vi "GenerateCode.vi"(0 "XRef":T17, 1 "Terms":T14, 2 "Diagram":T13, 3 "State In":T1) -> (14 "Generated Code?":T9, 15 "Reply":T12, 16 "Fatal Error Out":T11, 17 "State Out":T1)   [LabVIEW 2021, in "myRIO PWM Open.xnode"]
uses:
  <vilib>/myRIO/Instrument Drivers/Onboard IO/PWM/vis/myRIO PWM Open.xnode
  <vilib>/XNodeSupport/XNodeXNodeRef.ctl
  <vilib>/XNodeSupport/XNodeTermIDPairs.ctl
  <vilib>/XNodeSupport/XNodeTermIDPair.ctl
  <vilib>/XNodeSupport/XNodeTermRef.ctl
  <vilib>/XNodeSupport/XNodeString.ctl
  <vilib>/XNodeSupport/XNodeTopLevelDiagramRef.ctl
  <vilib>/myRIO/Instrument Drivers/Onboard IO/PWM/vis/State.ctl
  <vilib>/myRIO/Common/Instrument Driver Framework/Utilities/typedefs/myRIOXPeripheral.ctl
  <vilib>/XNodeSupport/XNodeTerm4Array.ctl
  <vilib>/XNodeSupport/XNodeTerm4.ctl
  <vilib>/XNodeSupport/XNodeVariant.ctl
  <vilib>/XNodeSupport/XNodeRect32.ctl
  <vilib>/XNodeSupport/XNodeInt.ctl
  <vilib>/XNodeSupport/XNodeBool.ctl
  <vilib>/XNodeSupport/XNodeTermDirection.ctl
  <vilib>/XNodeSupport/XNodeStringArray.ctl
  <vilib>/XNodeSupport/XNodeErrorCluster.ctl
  <vilib>/userdefined/High Color/nirio_resource_hc.ctl
  <vilib>/XNodeSupport/NI_XNodeSupport.lvlib
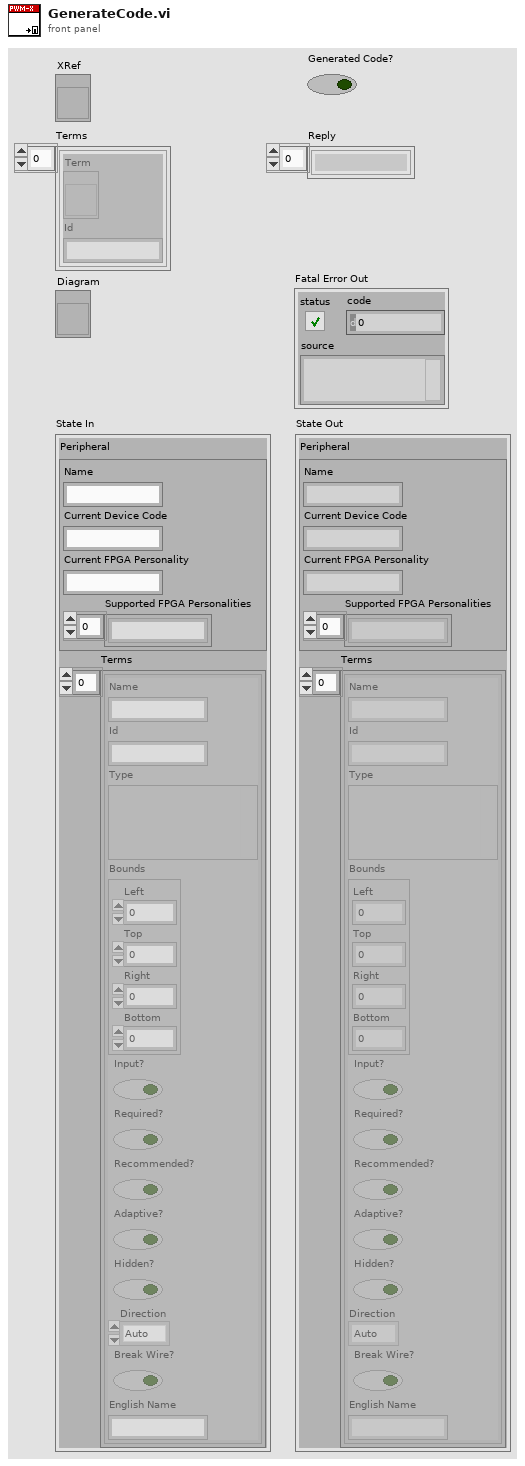
[diagram p1: front panel]
types:
  T1 = typedef "myRIO PWM Open.xnode/State.ctl" = cluster{"Peripheral":T2, "Terms":T3}
  T2 = typedef "myRIOXPeripheral.ctl" = cluster{"Name":string, "Current Device Code":string, "Current FPGA Personality":string, "Supported FPGA Personalities":string[]}
  T3 = typedef "NI_XNodeSupport.lvlib/XNodeTerm4Array.ctl" = T4[]
  T4 = typedef "NI_XNodeSupport.lvlib/XNodeTerm4.ctl" = cluster{"Name":T5, "Id":T5, "Type":T6, "Bounds":T7, "Input?":T9, "Required?":T9, "Recommended?":T9, "Adaptive?":T9, "Hidden?":T9, "Direction":T10, "Break Wire?":T9, "English Name":T5}
  T5 = typedef "NI_XNodeSupport.lvlib/XNodeString.ctl" = string
  T6 = typedef "NI_XNodeSupport.lvlib/XNodeVariant.ctl" = variant
  T7 = typedef "NI_XNodeSupport.lvlib/XNodeRect32.ctl" = cluster{"Left":T8, "Top":T8, "Right":T8, "Bottom":T8}
  T8 = typedef "NI_XNodeSupport.lvlib/XNodeInt.ctl" = i32
  T9 = typedef "NI_XNodeSupport.lvlib/XNodeBool.ctl" = bool
  T10 = typedef "NI_XNodeSupport.lvlib/XNodeTermDirection.ctl" = enum32{"Auto", "Up", "Down", "Left", "Right", "Center"}
  T11 = typedef "NI_XNodeSupport.lvlib/XNodeErrorCluster.ctl" = errorcluster
  T12 = typedef "NI_XNodeSupport.lvlib/XNodeStringArray.ctl" = T5[]
  T13 = typedef "NI_XNodeSupport.lvlib/XNodeTopLevelDiagramRef.ctl" = refnum<vi>
  T14 = typedef "NI_XNodeSupport.lvlib/XNodeTermIDPairs.ctl" = T15[]
  T15 = typedef "NI_XNodeSupport.lvlib/XNodeTermIDPair.ctl" = cluster{"Term":T16, "Id":T5}
  T16 = typedef "NI_XNodeSupport.lvlib/XNodeTermRef.ctl" = refnum<vi>
  T17 = typedef "NI_XNodeSupport.lvlib/XNodeXNodeRef.ctl" = refnum<vi>
  T18 = typedef "nirio_resource_hc.ctl" = tag
  T19 = typedef "LVPositionTypeDef.ctl" = cluster{"Left":i32, "Top":i32}
  T20 = typedef "Hardware Version Enum.ctl" = enum16{"Unknown", "myRIO-1900", "myRIO-1950", "roboRIO", "NI ELVIS RIO CM", "ELVIS III"}
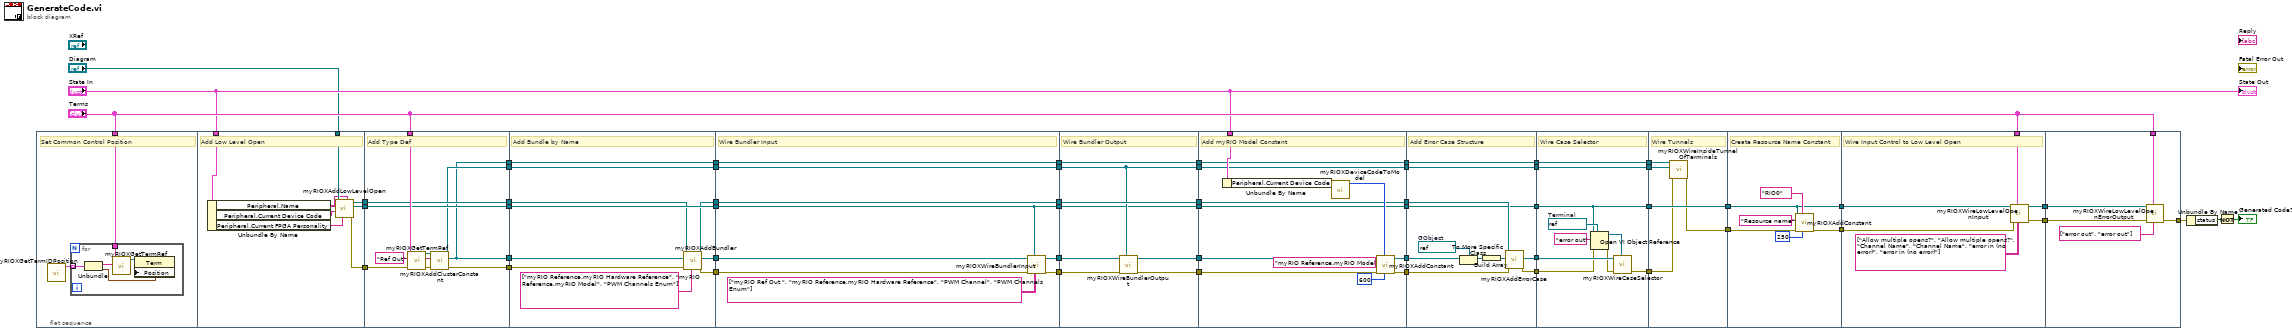
[diagram p0: block diagram]
diagram:
  n1 = flat-sequence {
    tunnel: "Terms" -> [w56]
    tunnel: "State In" -> [w69]
    tunnel: "Diagram" -> [w68]
    tunnel: [w67] -> w52
    tunnel: [w66] -> w48
    tunnel: [w64] -> w14
    tunnel: "Terms" -> [w79]
    tunnel: [w73] -> w54
    tunnel: [w76] -> w53
    tunnel: w52 -> [w76]
    tunnel: [w75] -> w49
    tunnel: w48 -> [w75]
    tunnel: [w74] -> w44
    tunnel: [w73] -> w39
    tunnel: [w72] -> w15
    tunnel: w14 -> [w71]
    tunnel: w54 -> [w89]
    tunnel: w53 -> [w86]
    tunnel: [w88] -> w51
    tunnel: [w87] -> w50
    tunnel: w49 -> [w87]
    tunnel: [w85] -> w46
    tunnel: w44 -> [w84]
    tunnel: [w84] -> w42
    tunnel: [w83] -> w40
    tunnel: w39 -> [w83]
    tunnel: w15 -> [w82]
    tunnel: [w81] -> w13
    tunnel: w51 -> [w98]
    tunnel: w50 -> [w93]
    tunnel: [w97] -> w38
    tunnel: [w96] -> w36
    tunnel: w46 -> [w96]
    tunnel: [w95] -> w34
    tunnel: w42 -> [w95]
    tunnel: [w94] -> w32
    tunnel: w40 -> [w94]
    tunnel: [w93] -> w29
    tunnel: w13 -> [w92]
    tunnel: [w91] -> w12
    tunnel: w38 -> [w106]
    tunnel: [w103] -> w37
    tunnel: w36 -> [w105]
    tunnel: [w105] -> w35
    tunnel: w34 -> [w102]
    tunnel: [w102] -> w33
    tunnel: w32 -> [w104]
    tunnel: [w104] -> w31
    tunnel: [w101] -> w30
    tunnel: w29 -> [w101]
    tunnel: w12 -> [w100]
    tunnel: [w99] -> w11
    tunnel: w37 -> [w119]
    tunnel: "State In" -> [w117]
    tunnel: [w113] -> w47
    tunnel: w35 -> [w113]
    tunnel: [w112] -> w45
    tunnel: [w111] -> w43
    tunnel: w33 -> [w111]
    tunnel: [w110] -> w41
    tunnel: w31 -> [w110]
    tunnel: w30 -> [w109]
    tunnel: [w109] -> w27
    tunnel: w11 -> [w108]
    tunnel: [w107] -> w10
    tunnel: w47 -> [w130]
    tunnel: w45 -> [w129]
    tunnel: [w125] -> w25
    tunnel: w43 -> [w125]
    tunnel: [w124] -> w23
    tunnel: w41 -> [w124]
    tunnel: [w123] -> w21
    tunnel: w27 -> [w123]
    tunnel: [w122] -> w19
    tunnel: w10 -> [w121]
    tunnel: [w120] -> w9
    tunnel: w25 -> [w140]
    tunnel: [w140] -> w24
    tunnel: w23 -> [w139]
    tunnel: [w139] -> w22
    tunnel: w21 -> [w135]
    tunnel: [w135] -> w20
    tunnel: w19 -> [w138]
    tunnel: w9 -> [w131]
    tunnel: [w133] -> w8
    tunnel: w24 -> [w144]
    tunnel: w22 -> [w145]
    tunnel: [w143] -> w28
    tunnel: w20 -> [w143]
    tunnel: w8 -> [w142]
    tunnel: [w141] -> w7
    tunnel: w28 -> [w148]
    tunnel: [w148] -> w26
    tunnel: w7 -> [w147]
    tunnel: [w146] -> w6
    tunnel: w26 -> [w155]
    tunnel: "Terms" -> [w156]
    tunnel: [w154] -> w18
    tunnel: [w153] -> w17
    tunnel: w6 -> [w152]
    tunnel: [w161] -> w3
    tunnel: w18 -> [w162]
    tunnel: w17 -> [w160]
    tunnel: "Terms" -> [w159]
    frame #0 {
      # "Set Common Control Position"
      n2 = call <vilib>:"myRIOXGetTermIDPosition.vi"() -> ("Term ID Postion"=w55:cluster{"Term ID":string, "Position":T19}[])  [unwired: 11 in]
      n3 = for {
        tunnel: w56 -> [w61]
        tunnel: w55 -> [w59] mode=indexing
        n4 = Unbundle(w59) -> ("Term ID"=w58:string, "Position"=w57:T19)
        n5 = call <vilib>:"myRIOXGetTermRef.vi"("Term ID"=w58, "Terms"=w61) -> ("Terminal Reference"=w60:T16)  [unwired: 7 in, 2 out]
        n6 = property class="Term"(reference=w60, "Position"=w57) -> ()  [unwired: 1 in, 2 out]
      }
    }
    frame #1 {
      # "Add Low Level Open"
      n7 = Unbundle By Name(w69) -> ("Peripheral.Name"=w62:string, "Peripheral.Current Device Code"=w65:string, "Peripheral.Current FPGA Personality"=w63:string)
      n8 = call <vilib>:"myRIOXAddLowLevelOpen.vi"("Peripheral Name"=w62, "FPGA Personality"=w63, "Device Code"=w65, "VI Name"=w62, "Diagram Reference"=w68) -> ("error out"=w64:errorcluster, "SubVI Reference"=w66:refnum<vi>, "Duplicated Diagram Reference"=w67:T13)  [unwired: 4 in]
    }
    frame #2 {
      # "Add Type Def"
      n9 = call <vilib>:"myRIOXGetTermRef.vi"("Term ID"="Ref Out", "Terms"=w79) -> ("Full Term ID"=w77:T5, "Terminal Reference"=w70:T16)  [unwired: 7 in, 1 out]
      n10 = call <vilib>:"myRIOXAddClusterConstant.vi"("error in (no error)"=w71, "Full Term ID"=w77, "Term Reference"=w70) -> ("error out"=w72:errorcluster, "Cluster Constant Terminal Reference"=w73:refnum<vi>, "Duplicated Term Reference"=w74:T16)  [unwired: 6 in]
    }
    frame #3 {
      # "Add Bundle by Name"
      n11 = call <vilib>:"myRIOXAddBundler.vi"("Element Names"=string[] ["myRIO Reference.myRIO Hardware Reference", "myRIO Reference.myRIO Model", "PWM Channels Enum"], "error in (no error)"=w82, "Cluster Constant Terminal Reference"=w89, "Diagram Reference"=w86) -> ("error out"=w81:errorcluster, "Named Bundler Reference"=w88:refnum<vi>, "Duplicated Diagram Reference"=w85:T13)  [unwired: 5 in]
    }
    frame #4 {
      # "Wire Bundler Input"
      n12 = call <vilib>:"myRIOXWireBundlerInput.vi"("Wiring Specs"=string[][] [["myRIO Ref Out ", "myRIO Reference.myRIO Hardware Reference"], ["PWM Channel", "PWM Channels Enum"]], "SubVI Reference"=w93, "error in (no error)"=w92, "Named Bundler Reference"=w98) -> ("error out"=w91:errorcluster, "Duplicated Named Bundler Reference"=w97:refnum<vi>)  [unwired: 6 in]
    }
    frame #5 {
      # "Wire Bundler Output"
      n13 = call <vilib>:"myRIOXWireBundlerOutput.vi"("Sink Terminam Reference"=w102, "error in (no error)"=w100, "Named Bundler Reference"=w106) -> ("error out"=w99:errorcluster, "Duplicated Named Bundler Reference"=w103:refnum<vi>)  [unwired: 7 in]
    }
    frame #6 {
      # "Add myRIO Model Constant"
      n14 = Unbundle By Name(w117) -> ("Peripheral.Current Device Code"=w116:string)
      n15 = call <vilib>:"myRIOXDeviceCodeToModel.vi"("Device Code"=w116) -> ("myRIO Reference.myRIO Model"=w115:T20)  [unwired: 10 in]
      n16 = call <vilib>:"myRIOXAddConstant.vi"("Left (0)"=600 ("Left"), "Value"=w115, "error in (no error)"=w108, "Terminal Name"="myRIO Reference.myRIO Model", "Owner Reference"=w119) -> ("error out"=w107:errorcluster, "Duplicated Owner Reference"=w112:refnum<vi>)  [unwired: 5 in]
    }
    frame #7 {
      w126 = refnum<vi> refnum  # GObject
      # "Add Error Case Structure"
      n17 = To More Specific Class(target class=w126, reference=w129) -> (specific class reference=w127:refnum<vi>)  [unwired: 1 in, 1 out]
      n18 = Build Array(w127) -> (w128:refnum<vi>[])
      n19 = call <vilib>:"myRIOXAddErrorCase.vi"("error in (no error)"=w121, "Enclosed Object References"=w128, "Diagram Reference"=w130) -> ("error out"=w120:errorcluster, "Case Structure Reference"=w122:refnum<vi>)  [unwired: 6 in, 1 out]
    }
    frame #8 {
      w137 = refnum<vi> refnum  # Terminal
      # "Wire Case Selector"
      n20 = Open VI Object Reference(7:w137, 8:w131, 10:"error out" ("name/order"), 11:w135) -> (0:w132:errorcluster, 3:w136:refnum<vi>)
      n21 = call <vilib>:"myRIOXWireCaseSelector.vi"("Source Terminam Reference"=w136, "error in (no error)"=w132, "Case Structure Reference"=w138) -> ("error out"=w133:errorcluster)  [unwired: 7 in, 1 out]
    }
    frame #9 {
      # "Wire Tunnels"
      n22 = call <vilib>:"myRIOXWireInsideTunnelOfTerminals.vi"("error in (no error)"=w142, "Sink Terminam Reference"=w144, "Source Terminam Reference"=w145) -> ("error out"=w141:errorcluster)  [unwired: 6 in, 2 out]
    }
    frame #10 {
      # "Create Resource Name Constant"
      n23 = call <vilib>:"myRIOXAddConstant.vi"("Left (0)"=250 ("Left"), "Value"=T18 "RIO0" ("Resource name"), "error in (no error)"=w147, "Terminal Name"="Resource name", "Owner Reference"=w148) -> ("error out"=w146:errorcluster)  [unwired: 5 in, 1 out]
    }
    frame #11 {
      # "Wire Input Control to Low Level Open"
      n24 = call <vilib>:"myRIOXWireLowLevelOpenInput.vi"("Wiring Specs"=string[][] [["Allow multiple opens?", "Allow multiple opens?"], ["Channel Name", "Channel Name"], ["error in (no error)", "error in (no error)"]], "Terms"=w156, "error in (no error)"=w152, "SubVI Reference"=w155) -> ("error out"=w154:errorcluster, "Duplicated SubVI Reference"=w153:refnum<vi>)  [unwired: 6 in]
    }
    frame #12 {
      n25 = call <vilib>:"myRIOXWireLowLevelOpenErrorOutput.vi"("Wiring Specs"=string[] ["error out", "error out"], "Terms"=w159, "error in (no error)"=w162, "SubVI Reference"=w160) -> ("error out"=w161:errorcluster)  [unwired: 6 in, 1 out]
    }
  }
  n26 = Unbundle By Name(w3) -> ("status"=w2:bool)
  n27 = Not(x=w2) -> (.not. x?=→"Generated Code?":bool)
  "State Out" <- "State In"
